vi "Create Hierarchy Table Row.vi"(8 "error in (no error)":errorcluster, 9 "data":T2, 10 "URL with params":string, 11 "Refnum in":T1) -> (0 "error out":errorcluster, 2 "OK":bool, 3 "Refnum out":T1)   [LabVIEW 2018]
uses:
  <vilib>/httpClient/ClientHandle.ctl
  <vilib>/httpClient/POSTBuffer.vi
  <vilib>/httpClient/LabVIEWHTTPClient.lvlib
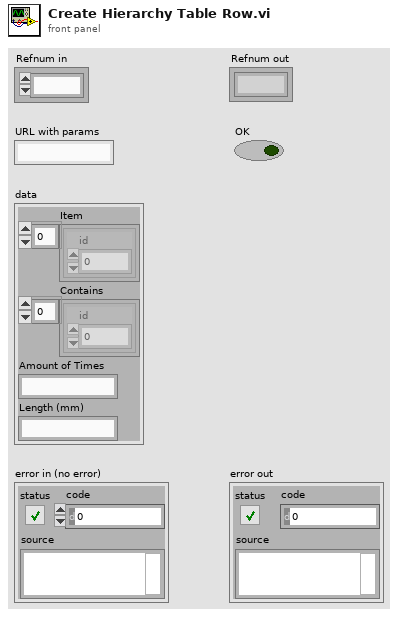
[diagram p1: front panel]
types:
  T1 = typedef "LabVIEWHTTPClient.lvlib/ClientHandle.ctl" = refnum<k1>
  T2 = cluster{"Item":cluster{"id":i32}[], "Contains":cluster{"id":i32}[], "Amount of Times":string, "Length (mm)":string}
  T3 = cluster{"ID":i32, "Item":cluster{"id":i32}[], "Contains":cluster{"id":i32}[], "Amount of Times":string, "Length (mm)":string}
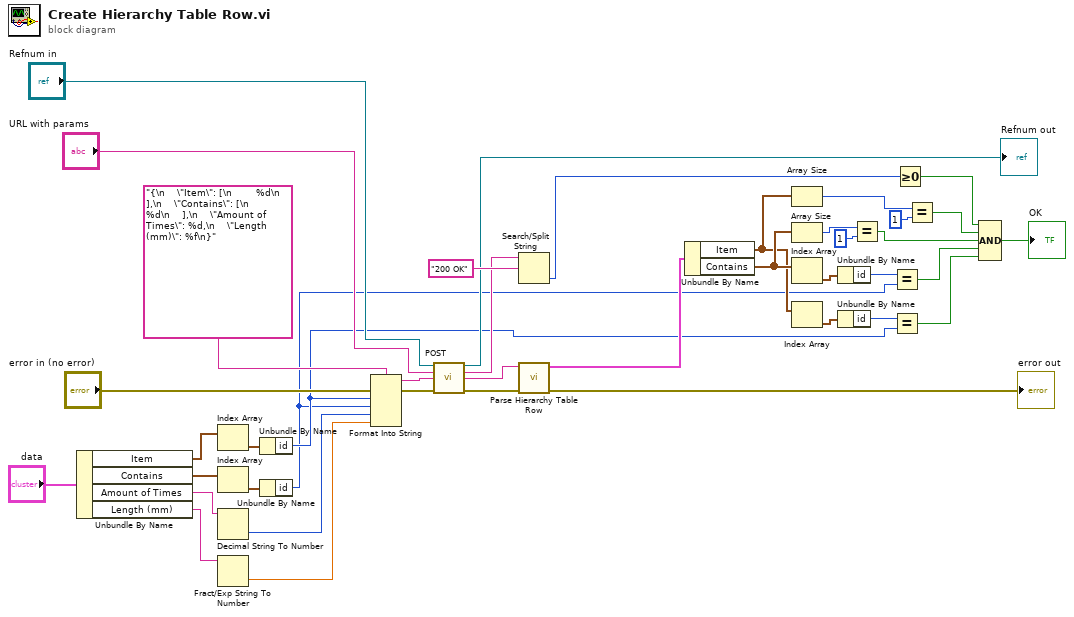
[diagram p0: block diagram]
diagram:
  n1 = Unbundle By Name("data") -> ("Item"=w11:cluster{"id":i32}[], "Contains"=w10:cluster{"id":i32}[], "Amount of Times"=w4:string, "Length (mm)"=w2:string)
  n2 = Index Array(array=w11) -> (element=w9:cluster{"id":i32})  [unwired: 1 in]
  n3 = Index Array(array=w10) -> (element=w7:cluster{"id":i32})  [unwired: 1 in]
  n4 = Decimal String To Number(string=w4) -> (number=w3:i32)  [unwired: 2 in, 1 out]
  n5 = Fract/Exp String To Number(string=w2) -> (number=w1:dbl)  [unwired: 3 in, 1 out]
  n6 = Unbundle By Name(w9) -> ("id"=w8:i32)
  n7 = Unbundle By Name(w7) -> ("id"=w5:i32)
  n8 = Format Into String(format string="{\n    \"Item\": [\n        %d\n    ],\n    \"Contains\": [\n        %d\n    ],\n    \"Amount of Times\": %d,\n    \"Length (mm)\": %f\n}" ("url"), error in="error in (no error)", w8, w5, w3, w1) -> (resulting string=w17:string, error out=w15:errorcluster)  [unwired: 1 in]
  n9 = call-poly <vilib>:"POST.vi"("client handle"="Refnum in", "url"="URL with params", "buffer"=w17, "error in (no error)"=w15) -> ("client handle out"=→"Refnum out":T1, "headers"=w20:string, "body"=w19:string, "error out"=w23:errorcluster)  [unwired: 8 in]
  n10 = Search/Split String(string=w20, search string/char (-)="200 OK") -> (offset of match=w22:i32)  [unwired: 1 in, 2 out]
  n11 = call "Parse Hierarchy Table Row.vi"("Error in"=w23, "Rows Array JSON"=w19) -> ("Error out"=→"error out":errorcluster, "data"=w25:T3)  [unwired: 8 in]
  n12 = Unbundle By Name(w25) -> ("Item"=w26:cluster{"id":i32}[], "Contains"=w31:cluster{"id":i32}[])
  n13 = Array Size(array=w26) -> (size(s)=w27:i32)
  n14 = Array Size(array=w31) -> (size(s)=w30:i32)
  n15 = Index Array(array=w31) -> (element=w33:cluster{"id":i32})  [unwired: 1 in]
  n16 = Index Array(array=w26) -> (element=w32:cluster{"id":i32})  [unwired: 1 in]
  n17 = Unbundle By Name(w33) -> ("id"=w37:i32)
  n18 = Unbundle By Name(w32) -> ("id"=w38:i32)
  n19 = Equal?(x=w30, y=1) -> (x = y?=w36:bool)
  n20 = Equal?(x=w37, y=w5) -> (x = y?=w39:bool)
  n21 = Equal?(x=w38, y=w8) -> (x = y?=w40:bool)
  n22 = Greater Or Equal To 0?(x=w22) -> (x >= 0?=w34:bool)
  n23 = Equal?(x=w27, y=1) -> (x = y?=w35:bool)
  n24 = Compound Arithmetic op=AND(w34, w35, w36, w39, w40) -> (→"OK":bool)
